vi "DMM_Measurement.vi"() -> ()   [LabVIEW 2014]
uses:
  DMMP.lvclass
panel:
  out "SampleNum":i32
  in  "Reference":dbl format="%#_13g"
  in  "StopRef":refnum<data-value>
  in  "Input DMMP":refnum<class "DMMP.lvclass">
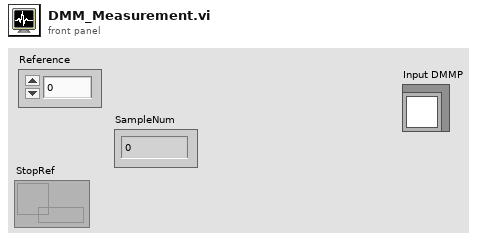
[diagram p1: front panel]
types:
  T1 = enum16{"open", "replace", "create", "open or create", "replace or create", "replace or create with confirmation"}
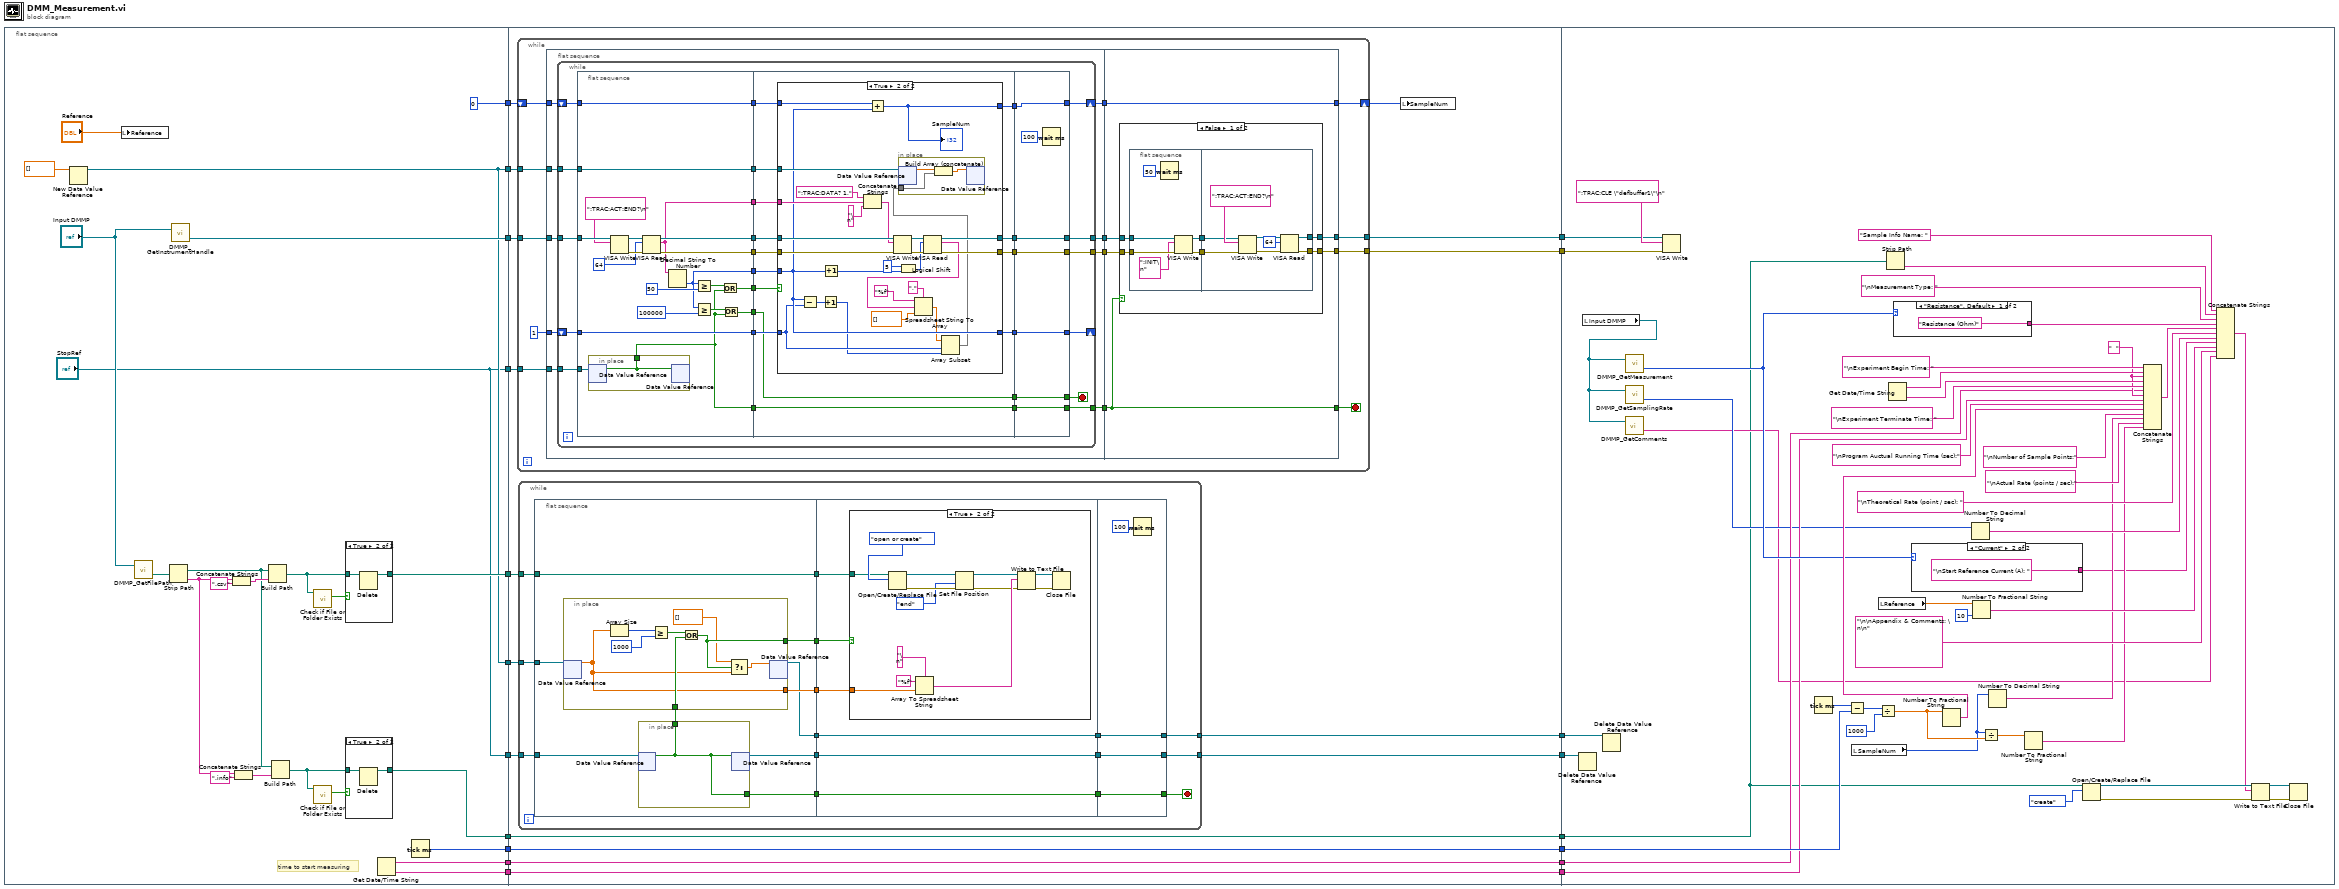
[diagram p0: block diagram]
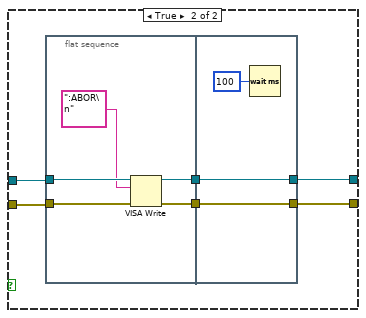
[diagram p6: hidden frame]
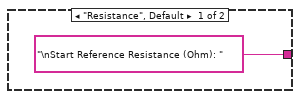
[diagram p7: hidden frame]
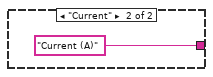
[diagram p8: hidden frame]
diagram:
  n1 = flat-sequence {
    tunnel: ["StopRef"] -> w19
    tunnel: [w28] -> w18
    tunnel: [0] -> w17
    tunnel: [w25] -> w16
    tunnel: [w26] -> w15
    tunnel: [w25] -> w14
    tunnel: ["StopRef"] -> w13
    tunnel: [w23] -> w12
    tunnel: [w22] -> w8
    tunnel: [w21] -> w7
    tunnel: [w20] -> w4
    tunnel: w19 -> [w64]
    tunnel: w18 -> [w63]
    tunnel: w17 -> [w62]
    tunnel: w16 -> [w61]
    tunnel: w15 -> [w60]
    tunnel: w14 -> [w59]
    tunnel: w13 -> [w58]
    tunnel: w12 -> [w57]
    tunnel: [w57] -> w11
    tunnel: [w56] -> w10
    tunnel: [w55] -> w9
    tunnel: w8 -> [w54]
    tunnel: w7 -> [w53]
    tunnel: [w54] -> w6
    tunnel: [w53] -> w5
    tunnel: w4 -> [w52]
    tunnel: [w52] -> w3
    tunnel: [w51] -> w2
    tunnel: [w50] -> w1
    tunnel: w11 -> [w285]
    tunnel: w10 -> [w332]
    tunnel: w9 -> [w331]
    tunnel: w6 -> [w291]
    tunnel: w5 -> [w290]
    tunnel: w3 -> [w329]
    tunnel: w2 -> [w325]
    tunnel: w1 -> [w324]
    frame #0 {
      # "time to start measuring"
      n2 = New Data Value Reference(data value=dbl[] []) -> (data value reference=w25:refnum<data-value>)  [unwired: 1 in, 1 out]
      n3 = local write "Reference"("Reference") -> ()
      n4 = call "DMMP_GetFilePath.vi"("Input DMMP"="Input DMMP") -> ("File Path"=w35:path)  [unwired: 1 in, 1 out]
      n5 = Strip Path(path=w35) -> (stripped path=w37:path, name=w39:string)
      n6 = call "DMMP_GetInstrumentHandle.vi"("Input DMMP"="Input DMMP") -> ("DMM Serial Port"=w28:refnum<visa-resource-name>)  [unwired: 1 in, 1 out]
      n7 = Concatenate Strings(w39, ".csv" ("string")) -> (w40:string)
      n8 = Concatenate Strings(w39, ".info" ("string")) -> (w36:string)
      n9 = Build Path(base path=w37, name or relative path=w40) -> (appended path=w33:path)
      n10 = Build Path(base path=w37, name or relative path=w36) -> (appended path=w31:path)
      n11 = call <vilib>:"Check if File or Folder Exists.vi"("path"=w33) -> ("file or folder exists?"=w34:bool)  [unwired: 8 in, 2 out]
      n12 = call <vilib>:"Check if File or Folder Exists.vi"("path"=w31) -> ("file or folder exists?"=w32:bool)  [unwired: 8 in, 2 out]
      n13 = case shown="True" w34 {
        tunnel: w33 -> [w46 w48]
        tunnel: [w46 w47] -> w26
        frame False {
        }
        frame True {
          n14 = Delete(path (use dialog)=w48) -> (deleted path=w47:path)  [unwired: 4 in, 2 out]
        }
      }
      n15 = case shown="True" w32 {
        tunnel: w31 -> [w43 w45]
        tunnel: [w43 w44] -> w23
        frame False {
        }
        frame True {
          n16 = Delete(path (use dialog)=w45) -> (deleted path=w44:path)  [unwired: 4 in, 2 out]
        }
      }
      n17 = Get Date/Time String() -> (date string=w22:string, time string=w21:string)  [unwired: 3 in]
      n18 = Tick Count (ms)() -> (millisecond timer value=w20:u32)
    }
    frame #1 {
      n19 = while {
        tunnel: w64 -> [w132]
        tunnel: w63 -> [w131]
        shift-right: [w123] -> w49
        shift-left: w62 -> [w130]
        tunnel: w61 -> [w129]
        tunnel: [w122] -> w51
        tunnel: [w121] -> w50
        stop <- w125 stop-if-true
        n20 = flat-sequence {
          tunnel: 1 -> [w142]
          tunnel: w132 -> [w141]
          tunnel: w131 -> [w140]
          tunnel: w130 -> [w139]
          tunnel: w129 -> [w138]
          tunnel: [w137] -> w128
          tunnel: [w136] -> w127
          tunnel: [w135] -> w126
          tunnel: [w134] -> w124
          tunnel: w128 -> [w250]
          tunnel: w127 -> [w249]
          tunnel: w126 -> [w248]
          tunnel: [w248] -> w125
          tunnel: [w247] -> w123
          tunnel: w124 -> [w247]
          tunnel: [w246] -> w122
          tunnel: [w245] -> w121
          frame #0 {
            n21 = while {
              shift-right: [w152] -> _
              shift-left: w142 -> [w158]
              tunnel: w141 -> [w169]
              tunnel: w140 -> [w168]
              shift-right: [w154] -> w134
              shift-left: w139 -> [w161]
              tunnel: w138 -> [w157]
              tunnel: [w147] -> w135
              tunnel: [w145] -> w137
              tunnel: [w143] -> w136
              stop <- w150 stop-if-true
              n22 = flat-sequence {
                tunnel: w169 -> [w189]
                tunnel: w168 -> [w188]
                tunnel: [w183] -> w167
                tunnel: [w182] -> w166
                tunnel: [w177] -> w165
                tunnel: [w176] -> w164
                tunnel: [w175] -> w163
                tunnel: [w174] -> w162
                tunnel: w161 -> [w173]
                tunnel: [w173] -> w160
                tunnel: [w172] -> w159
                tunnel: w158 -> [w172]
                tunnel: w157 -> [w171]
                tunnel: [w171] -> w156
                tunnel: [w170] -> w148
                tunnel: w167 -> [w201]
                tunnel: w166 -> [w200]
                tunnel: w165 -> [w204]
                tunnel: w164 -> [w194]
                tunnel: w163 -> [w203]
                tunnel: w162 -> [w202]
                tunnel: w160 -> [w199]
                tunnel: w159 -> [w198]
                tunnel: w156 -> [w197]
                tunnel: [w196] -> w155
                tunnel: [w195] -> w153
                tunnel: [w194] -> w151
                tunnel: [w193] -> w149
                tunnel: w148 -> [w193]
                tunnel: [w192] -> w146
                tunnel: [w191] -> w144
                tunnel: w155 -> [w244]
                tunnel: [w244] -> w154
                tunnel: w153 -> [w243]
                tunnel: [w243] -> w152
                tunnel: w151 -> [w241]
                tunnel: [w241] -> w150
                tunnel: [w240] -> w147
                tunnel: w149 -> [w240]
                tunnel: w146 -> [w239]
                tunnel: [w239] -> w145
                tunnel: [w238] -> w143
                tunnel: w144 -> [w238]
                frame #0 {
                  n23 = in-place {
                    in-place-border: [w190] -> w170
                    n24 = in-place-dvr #1(w189) -> (w190:bool)  [unwired: 1 out]
                    n25 = in-place-dvr #1(w190) -> ()  [unwired: 2 out]
                  }
                  n26 = VISA Write(VISA resource name=w188, write buffer=":TRAC:ACT:END?\n") -> (VISA resource name out=w186:refnum<visa-resource-name>, error out=w185:errorcluster)  [unwired: 1 in, 1 out]
                  n27 = VISA Read(VISA resource name=w186, byte count=u32 64, error in (no error)=w185) -> (VISA resource name out=w183:refnum<visa-resource-name>, read buffer=w175:string, error out=w182:errorcluster)  [unwired: 1 out]
                  n28 = Decimal String To Number(string=w175) -> (number=w174:i32)  [unwired: 2 in, 1 out]
                  n29 = Greater Or Equal?(x=w174, y=50) -> (x >= y?=w179:bool)
                  n30 = Greater Or Equal?(x=w174, y=100000) -> (x >= y?=w178:bool)
                  n31 = Or(x=w179, y=w170) -> (x .or. y?=w177:bool)
                  n32 = Or(x=w178, y=w170) -> (x .or. y?=w176:bool)
                }
                frame #1 {
                  n33 = case shown="True" w204 {
                    tunnel: w203 -> [_ w225]
                    tunnel: w202 -> [_ w213]
                    tunnel: w201 -> [w206 w232]
                    tunnel: w200 -> [w205 w231]
                    tunnel: w199 -> [w208 w234]
                    tunnel: w198 -> [w207 w211]
                    tunnel: w197 -> [_ w218]
                    tunnel: [w206 w221] -> w192
                    tunnel: [w205 w220] -> w191
                    tunnel: [w208 w219] -> w196
                    tunnel: [w207 w213] -> w195
                    frame False {
                    }
                    frame True {
                      n34 = Subtract(x=w213, y=w211) -> (x-y=w233:i32)
                      n35 = Increment(x=w233) -> (x+1=w210:i32)
                      n36 = Increment(x=w213) -> (x+1=w228:i32)
                      n37 = Concatenate Strings(":TRAC:DATA? 1," ("string"), w225, "\n" ("string")) -> (w222:string)
                      n38 = Add(x=w234, y=w213) -> (x+y=w219:i32)
                      "SampleNum" <- w219
                      n39 = VISA Write(VISA resource name=w232, write buffer=w222, error in (no error)=w231) -> (VISA resource name out=w230:refnum<visa-resource-name>, error out=w229:errorcluster)  [unwired: 1 out]
                      n40 = Logical Shift(y=i16 5, x=w228) -> (x << y=w226:i32)
                      n41 = VISA Read(VISA resource name=w230, byte count=w226, error in (no error)=w229) -> (VISA resource name out=w221:refnum<visa-resource-name>, read buffer=w214:string, error out=w220:errorcluster)  [unwired: 1 out]
                      n42 = Spreadsheet String To Array(delimiter (Tab)=",", format string="%f", spreadsheet string=w214, array type (2D Dbl)=dbl[] []) -> (array=w212:dbl[])
                      n43 = Array Subset(array=w212, index=w211, length=w210) -> (w209:dbl[])
                      n44 = in-place {
                        in-place-border: w209 -> [w237]
                        n45 = in-place-dvr #2(w218) -> (w236:dbl[])  [unwired: 1 out]
                        n46 = Build Array (concatenate)(w236, w237) -> (w235:dbl[])
                        n47 = in-place-dvr #2(w235) -> ()  [unwired: 2 out]
                      }
                    }
                  }
                }
                frame #2 {
                  n48 = Wait (ms)(milliseconds to wait=u32 100) -> ()  [unwired: 1 out]
                }
              }
            }
          }
          frame #1 {
            n49 = case shown="False" w248 {
              tunnel: w250 -> [w254 w274]
              tunnel: w249 -> [w253 w273]
              tunnel: [w252 w272] -> w246
              tunnel: [w251 w271] -> w245
              frame False {
                n50 = flat-sequence {
                  tunnel: w254 -> [w261]
                  tunnel: w253 -> [w260]
                  tunnel: [w258] -> w256
                  tunnel: [w257] -> w255
                  tunnel: w256 -> [w266]
                  tunnel: w255 -> [w265]
                  tunnel: [w264] -> w252
                  tunnel: [w263] -> w251
                  frame #0 {
                    n51 = Wait (ms)(milliseconds to wait=u32 50) -> ()  [unwired: 1 out]
                    n52 = VISA Write(VISA resource name=w261, write buffer=":INIT\n", error in (no error)=w260) -> (VISA resource name out=w258:refnum<visa-resource-name>, error out=w257:errorcluster)  [unwired: 1 out]
                  }
                  frame #1 {
                    n53 = VISA Write(VISA resource name=w266, write buffer=":TRAC:ACT:END?\n", error in (no error)=w265) -> (VISA resource name out=w269:refnum<visa-resource-name>, error out=w268:errorcluster)  [unwired: 1 out]
                    n54 = VISA Read(VISA resource name=w269, byte count=u32 64, error in (no error)=w268) -> (VISA resource name out=w264:refnum<visa-resource-name>, error out=w263:errorcluster)  [unwired: 2 out]
                  }
                }
              }
              frame True {
                n55 = flat-sequence {
                  tunnel: w274 -> [w281]
                  tunnel: w273 -> [w280]
                  tunnel: [w278] -> w276
                  tunnel: [w277] -> w275
                  tunnel: [w283] -> w272
                  tunnel: w276 -> [w283]
                  tunnel: [w282] -> w271
                  tunnel: w275 -> [w282]
                  frame #0 {
                    n56 = VISA Write(VISA resource name=w281, write buffer=":ABOR\n", error in (no error)=w280) -> (VISA resource name out=w278:refnum<visa-resource-name>, error out=w277:errorcluster)  [unwired: 1 out]
                  }
                  frame #1 {
                    n57 = Wait (ms)(milliseconds to wait=u32 100) -> ()  [unwired: 1 out]
                  }
                }
              }
            }
          }
        }
      }
      n58 = while {
        tunnel: w60 -> [w70]
        tunnel: w59 -> [w69]
        tunnel: w58 -> [w68]
        tunnel: [w67] -> w56
        tunnel: [w66] -> w55
        stop <- w65 stop-if-true
        n59 = flat-sequence {
          tunnel: w69 -> [w88]
          tunnel: w70 -> [w82]
          tunnel: [w87] -> w79
          tunnel: [w82] -> w78
          tunnel: [w85] -> w77
          tunnel: [w84] -> w76
          tunnel: [w83] -> w75
          tunnel: [w81] -> w74
          tunnel: w68 -> [w80]
          tunnel: w79 -> [w101]
          tunnel: w78 -> [w103]
          tunnel: w77 -> [w102]
          tunnel: [w98] -> w73
          tunnel: [w100] -> w72
          tunnel: w76 -> [w100]
          tunnel: [w99] -> w71
          tunnel: w75 -> [w99]
          tunnel: w74 -> [w98]
          tunnel: [w119] -> w65
          tunnel: w73 -> [w119]
          tunnel: [w118] -> w66
          tunnel: w72 -> [w118]
          tunnel: [w117] -> w67
          tunnel: w71 -> [w117]
          frame #0 {
            n60 = in-place {
              in-place-border: [w89] -> w86
              in-place-border: [w89] -> w81
              n61 = in-place-dvr #3(w80) -> (w89:bool)  [unwired: 1 out]
              n62 = in-place-dvr #3(w89) -> (w84:refnum<data-value>)  [unwired: 1 out]
            }
            n63 = in-place {
              in-place-border: [w93] -> w87
              in-place-border: w86 -> [w94]
              in-place-border: [w90] -> w85
              n64 = in-place-dvr #4(w88) -> (w90:dbl[])  [unwired: 1 out]
              n65 = Array Size(array=w90) -> (size(s)=w97:i32)
              n66 = Greater Or Equal?(x=w97, y=1000) -> (x >= y?=w95:bool)
              n67 = Or(x=w95, y=w94) -> (x .or. y?=w93:bool)
              n68 = Select(t=dbl[] [], s=w93, f=w90) -> (s? t:f=w91:dbl[])
              n69 = in-place-dvr #4(w91) -> (w83:refnum<data-value>)  [unwired: 1 out]
            }
          }
          frame #1 {
            n70 = case shown="True" w101 {
              tunnel: w103 -> [_ w111]
              tunnel: w102 -> [_ w116]
              frame False {
              }
              frame True {
                n71 = Open/Create/Replace File(file path (use dialog)=w111, operation (0:open)=T1."open or create") -> (refnum out=w108:refnum<file>, error out=w107:errorcluster)  [unwired: 4 in, 1 out]
                n72 = Array To Spreadsheet String(delimiter (Tab)="\n", array=w116, 3:"%f" ("format string")) -> (spreadsheet string=w113:string)
                n73 = Set File Position(refnum=w108, from (0:start)=enum16{"start", "end", "current"}."end", error in=w107) -> (refnum out=w105:refnum<file>, error out=w104:errorcluster)  [unwired: 1 in]
                n74 = Write to Text File(file (use dialog)=w105, text=w113, error in=w104) -> (refnum out=w110:refnum<file>, error out=w109:errorcluster)  [unwired: 1 in, 1 out]
                n75 = Close File(refnum=w110, error in=w109) -> ()  [unwired: 2 out]
              }
            }
          }
          frame #2 {
            n76 = Wait (ms)(milliseconds to wait=u32 100) -> ()  [unwired: 1 out]
          }
        }
      }
      n77 = local write "SampleNum"(w49) -> ()
    }
    frame #2 {
      w297 = "  " ("string")
      n78 = Delete Data Value Reference(data value reference=w331) -> ()  [unwired: 1 in, 2 out]
      n79 = local read "Input DMMP"() -> (w288:refnum<class "DMMP.lvclass">)
      n80 = Delete Data Value Reference(data value reference=w332) -> ()  [unwired: 1 in, 2 out]
      n81 = call "DMMP_GetComments.vi"("Input DMMP"=w288) -> ("Comments"=w287:string)  [unwired: 1 in, 1 out]
      n82 = call "DMMP_GetMeasurement.vi"("Input DMMP"=w288) -> ("Measurement"=w292:enum16{"Resistance", "Current"})  [unwired: 1 in, 1 out]
      n83 = call "DMMP_GetSamplingRate.vi"("Input DMMP"=w288) -> ("Sampling Rate (point / sec)"=w289:u32)  [unwired: 1 in, 1 out]
      n84 = VISA Write(VISA resource name=w325, write buffer=":TRAC:CLE \"defbuffer1\"\n", error in (no error)=w324) -> ()  [unwired: 3 out]
      n85 = Tick Count (ms)() -> (millisecond timer value=w330:u32)
      n86 = Subtract(x=w330, y=w329) -> (x-y=w328:u32)
      n87 = local read "SampleNum"() -> (w286:i32)
      n88 = local read "Reference"() -> (w313:dbl)
      n89 = Divide(x=w328, y=u32 1000) -> (x/y=w293:dbl)
      n90 = Strip Path(path=w285) -> (name=w321:string)  [unwired: 1 out]
      n91 = Get Date/Time String() -> (date string=w319:string, time string=w318:string)  [unwired: 3 in]
      n92 = case shown="\"Resistance\", Default" w292 {
        tunnel: ["Resistance (Ohm)" ("string") "Current (A)" ("string")] -> w295
        frame "Resistance", Default {
        }
        frame "Current" {
        }
      }
      n93 = case shown="\"Current\"" w292 {
        tunnel: ["\nStart Reference Resistance (Ohm): " "\nStart Reference Current (A): "] -> w294
        frame "Resistance", Default {
        }
        frame "Current" {
        }
      }
      n94 = Number To Fractional String(number=w293) -> (F-format string=w302:string)  [unwired: 3 in]
      n95 = Number To Decimal String(number=w289) -> (decimal integer string=w314:string)  [unwired: 1 in]
      n96 = Number To Fractional String(number=w313, precision (6)=i16 10) -> (F-format string=w311:string)  [unwired: 2 in]
      n97 = Divide(x=w286, y=w293) -> (x/y=w301:dbl)
      n98 = Number To Decimal String(number=w286) -> (decimal integer string=w299:string)  [unwired: 1 in]
      n99 = Number To Fractional String(number=w301) -> (F-format string=w300:string)  [unwired: 3 in]
      n100 = Open/Create/Replace File(file path (use dialog)=w285, operation (0:open)=T1."create") -> (refnum out=w309:refnum<file>, error out=w308:errorcluster)  [unwired: 4 in, 1 out]
      n101 = Concatenate Strings("\nExperiment Begin Time: ", w319, w297, w318, "\nExperiment Terminate Time: " ("string"), w291, w297, w290, "\nProgram Auctual Running Time (sec):" ("string"), w302, "\nNumber of Sample Points:" ("string"), w299, "\nActual Rate (points / sec):" ("string"), w300) -> (w317:string)
      n102 = Concatenate Strings("Sample Info Name: ", w321, "\nMeasurement Type: ", w295, w317, "\nTheoretical Rate (point / sec): ", w314, w294, w311, "\n\nAppendix & Comments: \n\n", w287) -> (w307:string)
      n103 = Write to Text File(file (use dialog)=w309, text=w307, error in=w308) -> (refnum out=w306:refnum<file>, error out=w305:errorcluster)  [unwired: 1 in, 1 out]
      n104 = Close File(refnum=w306, error in=w305) -> ()  [unwired: 2 out]
    }
  }
